vi "Reserve Shooter.vi"(7 "Description":string="Reserve", 8 "Command Info":T1, 10 "Command Name":string) -> (0 "Command Info":T1)   [LabVIEW 2025]
uses:
  <vilib>/Rock Robotics/WPI/Framework/Command Status Info.ctl
  <vilib>/Rock Robotics/WPI/Framework/Completion Status.ctl
  <vilib>/Rock Robotics/WPI/Framework/Completion Notifier.ctl
  Implementation/Shooter Setpoints.ctl
  Implementation/Shooter Operations.ctl
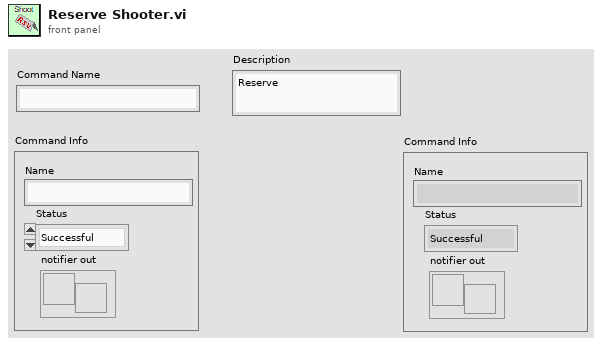
[diagram p1: front panel]
types:
  T1 = typedef "Command Status Info.ctl" = cluster{"Name":string, "Status":T2, "notifier out":T3}
  T2 = typedef "Completion Status.ctl" = enum16{"Successful", "Aborted", "Incomplete"}
  T3 = typedef "Completion Notifier.ctl" = refnum<notifier>
  T4 = typedef "Shooter Setpoints.ctl" = cluster{"Operation":T5, "Flywheel Setpoint":dbl, "Duration":dbl, "Kicker Setpoint":dbl, "Transfer 1 Setpoint":dbl, "Transfer 2 Setpoint":dbl, "Hood Setpoint":dbl}
  T5 = typedef "Shooter Operations.ctl" = enum16{"Reserve", "Read Current", "Immediate"}
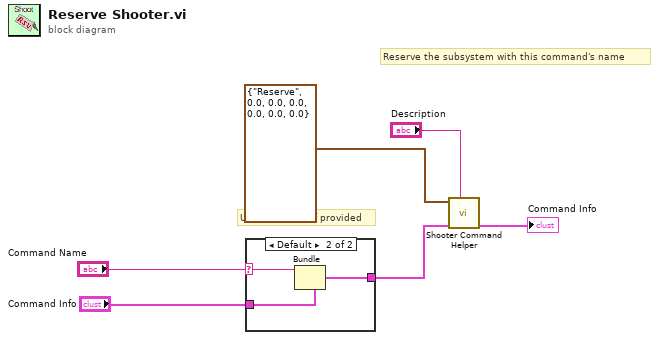
[diagram p0: block diagram]
diagram:
  # "Update name, if provided"
  # "Reserve the subsystem with this command's name"
  n1 = case shown="Default" "Command Name" {
    selector: "Command Name" -> [_ w8]
    tunnel: "Command Info" -> [w7 w10]
    tunnel: [w7 w9] -> w3
    frame "" {
    }
    frame Default {
      n2 = Bundle(cluster=w10, "Name"=w8) -> (w9:T1)  [unwired: 2 in]
    }
  }
  n3 = call "Shooter Command Helper.vi"("Description"="Description", "Command Info In"=w3, "SubSystem Data"=T4 {"Operation"=enum."Reserve", "Flywheel Setpoint"=0.0, "Duration"=0.0, "Kicker Setpoint"=0.0, "Transfer 1 Setpoint"=0.0, "Transfer 2 Setpoint"=0.0, "Hood Setpoint"=0.0}) -> ("Command Info Out"=→"Command Info":T1)  [unwired: 6 in, 2 out]
